vi "Check mtcdt temp.vi"(6 "VISA resource name":refnum<visa-resource-name>="COM5", 7 "Passed so far":bool, 8 "error in (no error)":errorcluster) -> (0 "error out":errorcluster, 2 "Response":string, 3 "Keyword found index":i32, 4 "VISA Refnum out":refnum<visa-resource-name>, 5 "Passed?":bool)   [LabVIEW 2024]
panel:
  out "output decimal line":string
  out "Keyword found":string
  in  "Wait for keywords":string[](array[string])=["5", "4", "3", "2"]
  in  "write buffer":string="cat /sys/class/hwmon/hwmon0/temp1_input\n"
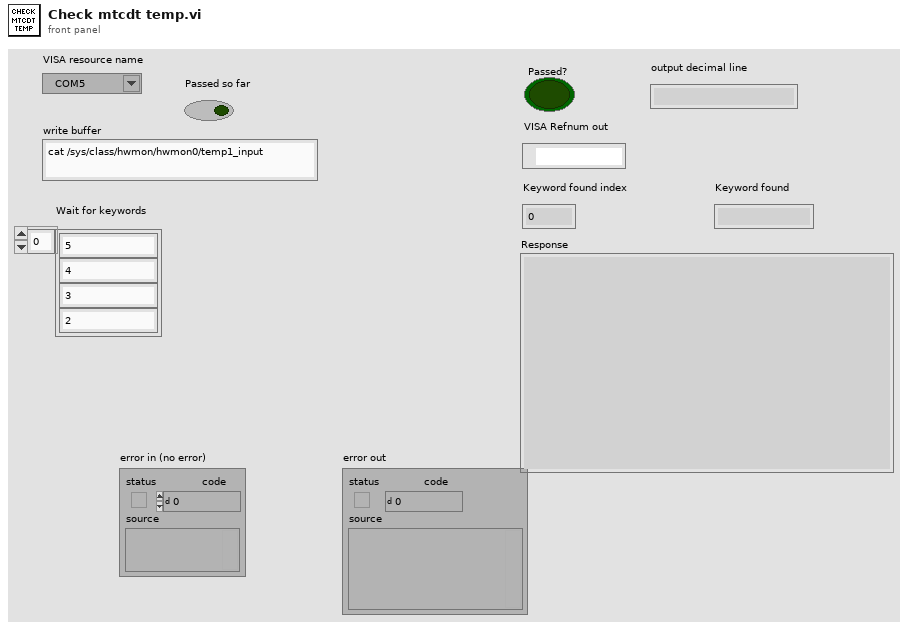
[diagram p1: front panel]
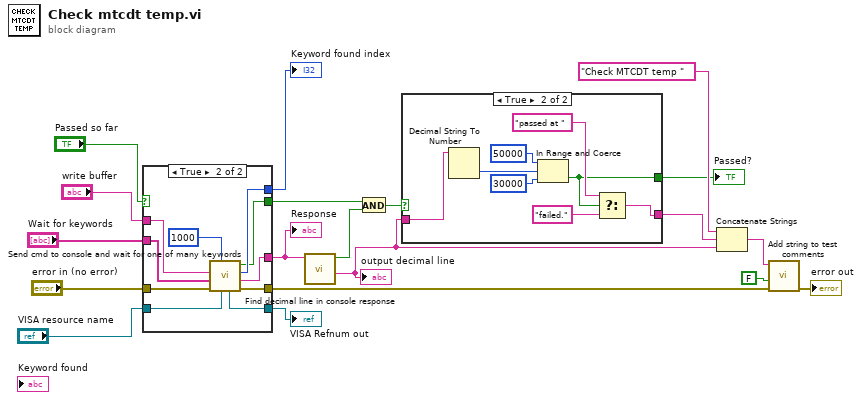
[diagram p0: block diagram]
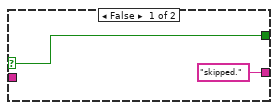
[diagram p2: hidden frame]
diagram:
  n1 = case shown="True" "Passed so far" {
    selector: "Passed so far" -> [w22 _]
    tunnel: "error in (no error)" -> [w21 w32]
    tunnel: [w21 w31] -> w11
    tunnel: "VISA resource name" -> [w20 w25]
    tunnel: "write buffer" -> [_ w30]
    tunnel: "Wait for keywords" -> [_ w29]
    tunnel: [w22 w23] -> w6
    tunnel: [_ w27] -> w8
    tunnel: [_ w26] -> w7
    tunnel: [w20 w24] -> w15
    frame False {
    }
    frame True {
      n2 = call "Send cmd to console and wait for one of many keywords.vi"("VISA resource name"=w25, "Timeout (1000 mSecs)"=u32 1000 ("Timeout (mSecs)"), "error in (no error)"=w32, "Wait for keywords"=w29, "write buffer"=w30) -> ("error out"=w31:errorcluster, "Response"=w26:string, "Keyword found index"=w27:i32, "Found key?"=w23:bool, "VISA Refnum out"=w24:refnum<visa-resource-name>)  [unwired: 2 in]
    }
  }
  "Keyword found index" <- w8
  "Response" <- w7
  "VISA Refnum out" <- w15
  n3 = call "Find decimal line in console response.vi"("Console response in"=w7) -> ("output decimal line"=w3:string, "Found decimal line"=w5:bool)  [unwired: 7 in, 2 out]
  "output decimal line" <- w3
  n4 = And(x=w6, y=w5) -> (x .and. y?=w4:bool)
  n5 = case shown="True" w4 {
    selector: w4 -> [w34 _]
    tunnel: w3 -> [_ w42]
    tunnel: [w34 w35] -> w2
    tunnel: ["skipped." w36] -> w1
    frame False {
    }
    frame True {
      n6 = Decimal String To Number(string=w42) -> (number=w41:i32)  [unwired: 2 in, 1 out]
      n7 = In Range and Coerce(upper limit=50000, x=w41, lower limit=30000) -> (In Range?=w35:bool)  [unwired: 1 out]
      n8 = Select(t="passed at ", s=w35, f="failed.") -> (s? t:f=w36:string)
    }
  }
  "Passed?" <- w2
  n9 = Concatenate Strings("Check MTCDT temp " ("string"), w1, w3) -> (w13:string)
  n10 = call "Add string to test comments.vi"("error in (no error)"=w11, "New Section (y)?"=FALSE, "Comments"=w13) -> ("error out"=→"error out":errorcluster)  [unwired: 7 in, 1 out]
